vi "eval_demo.vi"() -> ()   [LabVIEW 2021]
panel:
  out "value":dbl
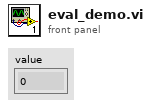
[diagram p1: front panel]
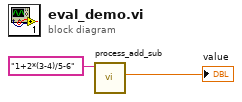
[diagram p0: block diagram]
diagram:
  n1 = call "process_add_sub.vi"("expression"="1+2*(3-4)/5-6") -> ("value"=→"value":dbl)  [unwired: 8 in, 1 out]
